vi "diody.vi"(3 "Akcja":T2, 5 "Wejście":T1) -> (2 "Wyjście":T1)   [LabVIEW 2014]
uses:
  AkcjaGFV.ctl
  diodyVIs/Diody_zbior.ctl
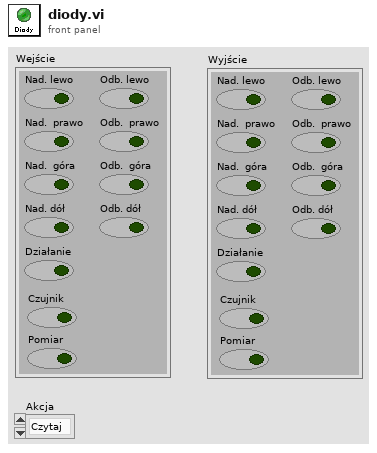
[diagram p1: front panel]
types:
  T1 = typedef "Diody_zbior.ctl" = cluster{"Nad. lewo":bool, "Nad.  prawo":bool, "Nad.  góra":bool, "Nad. dół":bool, "Działanie":bool, "Czujnik":bool, "Pomiar":bool, "Odb. dół":bool, "Odb.  góra":bool, "Odb.  prawo":bool, "Odb. lewo":bool}
  T2 = typedef "AkcjaGFV.ctl" = enum16{"Czytaj", "Zapisz", "Reset"}
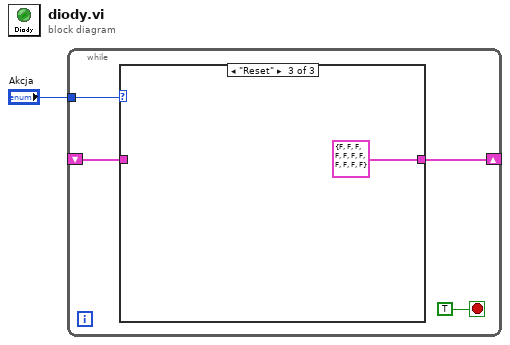
[diagram p0: block diagram]
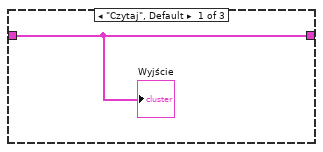
[diagram p2: hidden frame]
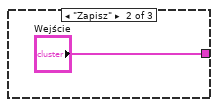
[diagram p3: hidden frame]
diagram:
  n1 = while {
    tunnel: "Akcja" -> [w5]
    shift-right: [w2] -> _
    shift-left: _ -> [w4]
    stop <- TRUE stop-if-true
    n2 = case shown="\"Reset\"" w5 {
      tunnel: w4 -> [w6 _ _]
      tunnel: [w6 "Wejście" T1 {"Nad. lewo"=FALSE, "Nad.  prawo"=FALSE, "Nad.  góra"=FALSE, "Nad. dół"=FALSE, "Działanie"=FALSE, "Czujnik"=FALSE, "Pomiar"=FALSE, "Odb. dół"=FALSE, "Odb.  góra"=FALSE, "Odb.  prawo"=FALSE, "Odb. lewo"=FALSE} ("Wejście")] -> w2
      frame "Czytaj", Default {
        "Wyjście" <- w6
      }
      frame "Zapisz" {
      }
      frame "Reset" {
      }
    }
  }
